vi "LabViewScanResultParser.vi"(0 "DataIn(str)":string, 1 "Limits_in":string[](array[string]), 7 "Comment":string, 11 "error in":errorcluster, 12 "FromDataFile(t)":bool, 13 "MSN":string) -> (2 "pass(ary)":bool[](array[boolean]), 4 "Pass?(T)":bool=TRUE, 6 "DataToResultFile":string[][](array[string]), 15 "error out":errorcluster)   [LabVIEW 2018]
panel:
  out "Array 3":string[](array[string])
  out "subarray 2":string[](array[string])
  out "P/F":string[](array[string])
  out "freq_mhz":string[](array[string])
  out "ampl_dB":string[](array[string])
  out "RxAnt":string[](array[string])
  out "TxAnt":string[](array[string])
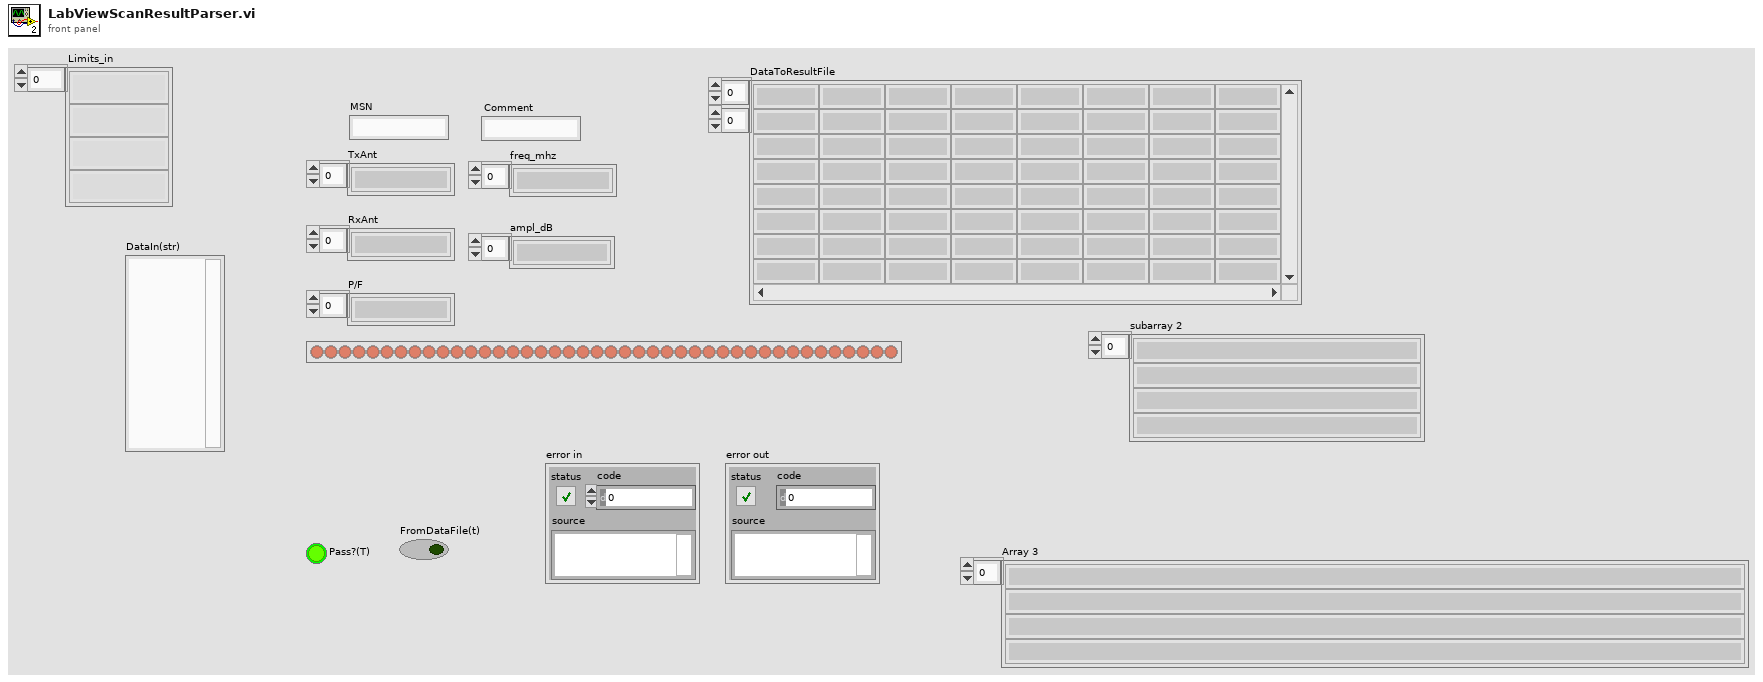
[diagram p1: front panel]
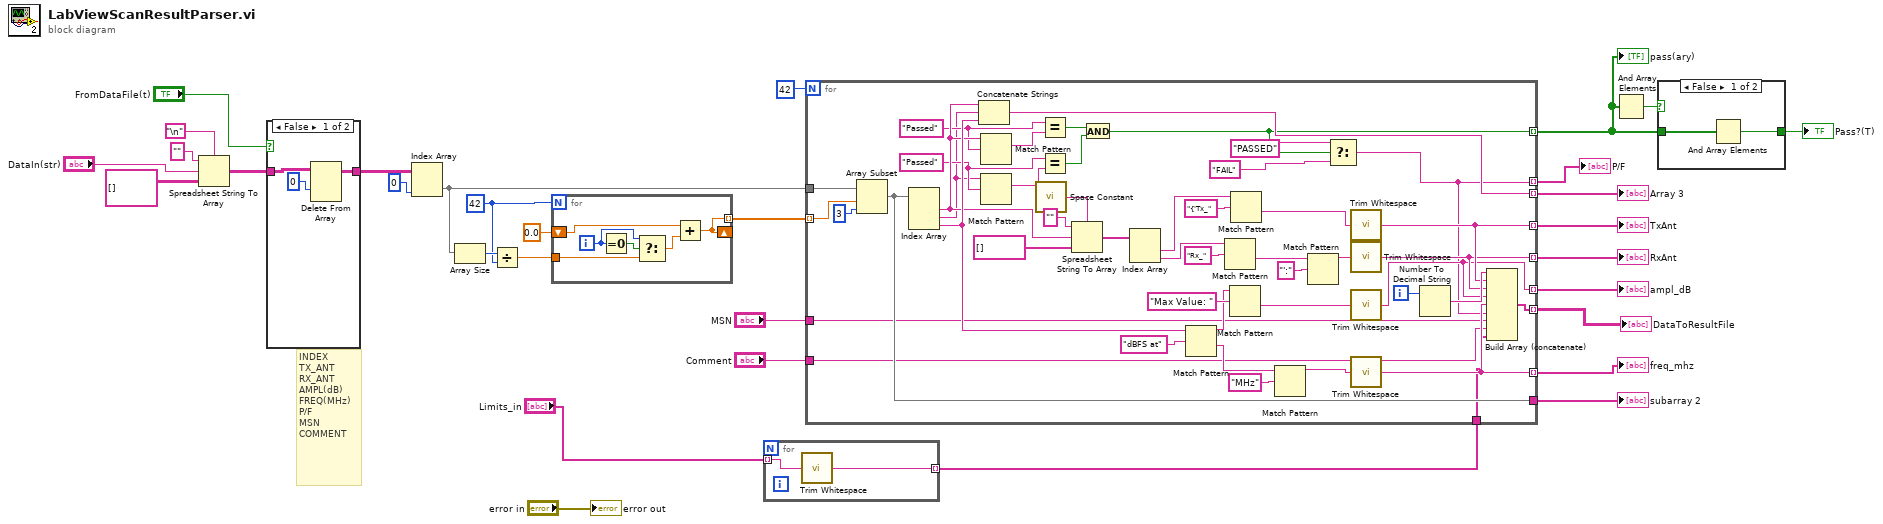
[diagram p0: block diagram]
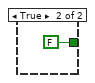
[diagram p2: hidden frame]
diagram:
  w24 = 42 ("y")
  # "INDEX\nTX_ANT\nRX_ANT\nAMPL(dB)\nFREQ(MHz)\nP/F\nMSN\nCOMMENT"
  n1 = Spreadsheet String To Array(delimiter (Tab)="\n", format string="", spreadsheet string="DataIn(str)", array type (2D Dbl)=string[][] []) -> (array=w29:string[][])
  n2 = case shown="False" "FromDataFile(t)" {
    tunnel: w29 -> [w34 w35]
    tunnel: [w32 w35] -> w21
    frame False {
      n3 = Delete From Array(array=w34, index (row)=0) -> (array with subset deleted=w32:string[][])  [unwired: 2 in, 1 out]
    }
    frame True {
    }
  }
  n4 = Index Array(array=w21, index (col)=0 ("disabled index (col)")) -> (element=w20:string[])  [unwired: 1 in]
  n5 = Array Size(array=w20) -> (size(s)=w25:i32)
  n6 = Divide(x=w25, y=w24) -> (x/y=w23:dbl)
  n7 = for {
    N: w24 -> [_]
    tunnel: w23 -> [w39]
    shift-right: [w36] -> _
    shift-left: 0.0 ("x+y") -> [w37]
    tunnel: [w36] -> w18 mode=indexing
    i -> [w38]
    n8 = Equal To 0?(x=w38) -> (x = 0?=w40:bool)
    n9 = Select(t=w38, s=w40, f=w39) -> (s? t:f=w41:dbl)
    n10 = Add(x=w37, y=w41) -> (x+y=w36:dbl)
  }
  n11 = for {
    tunnel: [w43] -> w2 mode=indexing
    tunnel: "Limits_in" -> [w42] mode=indexing
    n12 = call <vilib>:"Trim Whitespace.vi"("string"=w42) -> ("trimmed string"=w43:string)  [unwired: 1 in]
  }
  n13 = for {
    N: 42 -> [_]
    tunnel: w20 -> [w90]
    tunnel: [w87] -> w19
    tunnel: w18 -> [w88] mode=indexing
    tunnel: [w86] -> w17 mode=indexing
    tunnel: [w53] -> w15 mode=indexing
    tunnel: [w52] -> w14 mode=indexing
    tunnel: [w55] -> w13 mode=indexing
    tunnel: [w54] -> w12 mode=indexing
    tunnel: [w47] -> w9 mode=indexing
    tunnel: [w44] -> w8 mode=indexing
    tunnel: "MSN" -> [w51]
    tunnel: "Comment" -> [w50]
    tunnel: [w49] -> w5 mode=indexing
    tunnel: w2 -> [w48]
    i -> [w57]
    w61 = "Passed" ("regular expression")
    w64 = "Passed" ("regular expression")
    n14 = Array Subset(array=w90, index=w88, length=3) -> (w87:string[])
    n15 = Index Array(array=w87) -> (element #1=w65:string, element #2=w60:string, element #3=w85:string)  [unwired: 3 in]
    n16 = Concatenate Strings(w65, w60, w85) -> (w86:string)
    n17 = Match Pattern(string=w65, regular expression=w64) -> (match substring=w63:string)  [unwired: 1 in, 3 out]
    n18 = Match Pattern(string=w60, regular expression=w61) -> (match substring=w62:string)  [unwired: 1 in, 3 out]
    n19 = call <vilib>:"Space Constant.vi"() -> ("String"=w76:string)
    n20 = Equal?(x=w64, y=w63) -> (x = y?=w59:bool)
    n21 = Equal?(x=w61, y=w62) -> (x = y?=w58:bool)
    n22 = Spreadsheet String To Array(delimiter (Tab)=w76, format string="", spreadsheet string=w65, array type (2D Dbl)=string[] []) -> (array=w74:string[])
    n23 = And(x=w59, y=w58) -> (x .and. y?=w47:bool)
    n24 = Index Array(array=w74) -> (element #1=w73:string, element #2=w70:string)  [unwired: 2 in]
    n25 = Match Pattern(string=w85, regular expression="dBFS at") -> (before substring=w78:string, after substring=w83:string)  [unwired: 1 in, 2 out]
    n26 = Match Pattern(string=w70, regular expression="Rx_") -> (after substring=w68:string)  [unwired: 1 in, 3 out]
    n27 = Match Pattern(string=w78, regular expression="Max Value: " ("string")) -> (after substring=w81:string)  [unwired: 1 in, 3 out]
    n28 = Match Pattern(string=w73, regular expression="{'Tx_") -> (after substring=w71:string)  [unwired: 1 in, 3 out]
    n29 = Match Pattern(string=w83, regular expression="MHz") -> (before substring=w80:string)  [unwired: 1 in, 3 out]
    n30 = Match Pattern(string=w68, regular expression="':") -> (before substring=w66:string)  [unwired: 1 in, 3 out]
    n31 = Select(t="PASSED", s=w47, f="FAIL") -> (s? t:f=w44:string)
    n32 = call <vilib>:"Trim Whitespace.vi"("string"=w71) -> ("trimmed string"=w55:string)  [unwired: 1 in]
    n33 = call <vilib>:"Trim Whitespace.vi"("string"=w66) -> ("trimmed string"=w54:string)  [unwired: 1 in]
    n34 = call <vilib>:"Trim Whitespace.vi"("string"=w81) -> ("trimmed string"=w53:string)  [unwired: 1 in]
    n35 = call <vilib>:"Trim Whitespace.vi"("string"=w80) -> ("trimmed string"=w52:string)  [unwired: 1 in]
    n36 = Number To Decimal String(number=w57) -> (decimal integer string=w56:string)  [unwired: 1 in]
    n37 = Build Array (concatenate)(w56, w55, w54, w53, w52, w44, w51, w50, w48) -> (w49:string[])
  }
  "subarray 2" <- w19
  "Array 3" <- w17
  "ampl_dB" <- w15
  "freq_mhz" <- w14
  "TxAnt" <- w13
  "RxAnt" <- w12
  "pass(ary)" <- w9
  "P/F" <- w8
  "DataToResultFile" <- w5
  n38 = And Array Elements(Boolean array=w9) -> (logical AND=w10:bool)
  n39 = case shown="False" w10 {
    tunnel: [w92 FALSE] -> w11
    tunnel: w9 -> [w91 _]
    frame False {
      n40 = And Array Elements(Boolean array=w91) -> (logical AND=w92:bool)
    }
    frame True {
    }
  }
  "Pass?(T)" <- w11
  "error out" <- "error in"
